vi "Load API Tester--helper.vi"(8 "error in (no error)":errorcluster, 11 "Module DQMH Path":path) -> (0 "error out":errorcluster)   [LabVIEW 2020, in "UI Manager.lvlib"]
doc: "Opens a reference to a module's API Tester VI and runs it asynchronously.\n\nBeware: Rework the API Tester so it doesn't stop the module once it's closed!\n\n____\nHAMPEL SOFTWARE ENGINEERING v2.6.0 (2023-12-19 10:54)"
uses:
  UI Manager.lvlib
  Libraries/hse-libraries/Source/hse-dqmh/hse-dqmh-dynamicrequesters.lvlib
  Libraries/hse-libraries/Source/hse-dqmh/hse-dqmh.lvlib
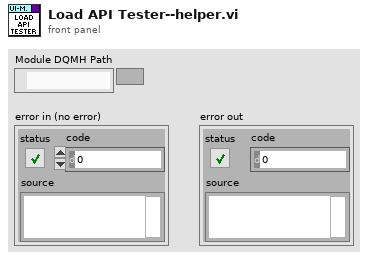
[diagram p1: front panel]
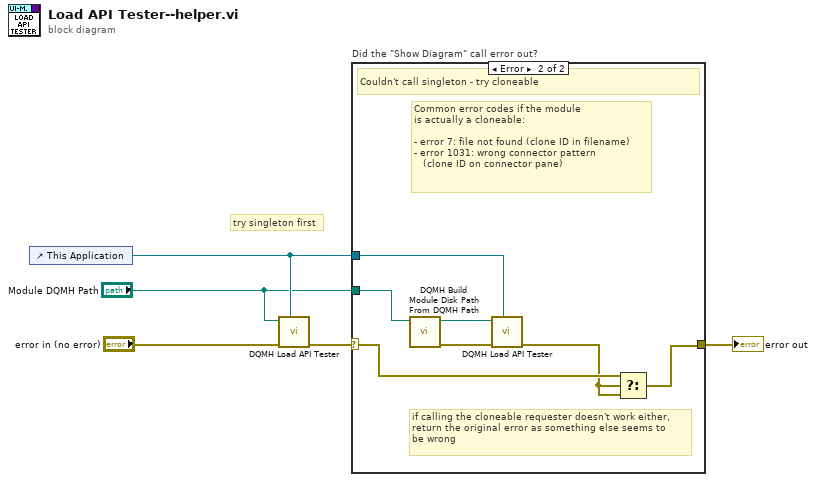
[diagram p0: block diagram]
diagram:
  # "try singleton first"
  n1 = control-ref of="This Application"() -> (w2:refnum<vi>)
  n2 = call "DQMH Load API Tester.vi"("Application reference"=w2, "error in (no error)"="error in (no error)", "Module Disk Path"="Module DQMH Path") -> ("error out"=w4:errorcluster)  [unwired: 8 in]
  n3 = case "Did the \"Show Diagram\" call error out?" shown="Error" w4 {
    selector: w4 -> [w6 w12]
    tunnel: "Module DQMH Path" -> [_ w13]
    tunnel: w2 -> [_ w10]
    tunnel: [w6 w11] -> w3
    frame No Error {
    }
    frame Error {
      # "if calling the cloneable requester doesn't work either,\nreturn the original error as something else seems to \nbe wrong"
      # "Common error codes if the module \nis actually a cloneable:\n\n- error 7: file not found (clone ID in filename)\n- error 1031: wrong connector pattern \n   (clone ID on connector pane)"
      # "Couldn't call singleton - try cloneable"
      n4 = call "DQMH Build Module Disk Path From DQMH Path.vi"("Module DQMH Path"=w13) -> ("error out"=w8:errorcluster, "Module Disk Path"=w9:path)  [unwired: 7 in, 2 out]
      n5 = call "DQMH Load API Tester.vi"("Application reference"=w10, "error in (no error)"=w8, "Module Disk Path"=w9) -> ("error out"=w7:errorcluster)  [unwired: 8 in]
      n6 = Select(t=w12, s=w7, f=w7) -> (s? t:f=w11:errorcluster)
    }
  }
  "error out" <- w3
